vi "NOT4.vi"(1 "A":bool[](array[boolean])=[FALSE, FALSE, FALSE, FALSE, FALSE, FALSE, FALSE, FALSE, FALSE, FALSE, FALSE, FALSE, FALSE, FALSE, FALSE, FALSE]) -> (0 "z":bool[](array[boolean]))   [LabVIEW 2012]
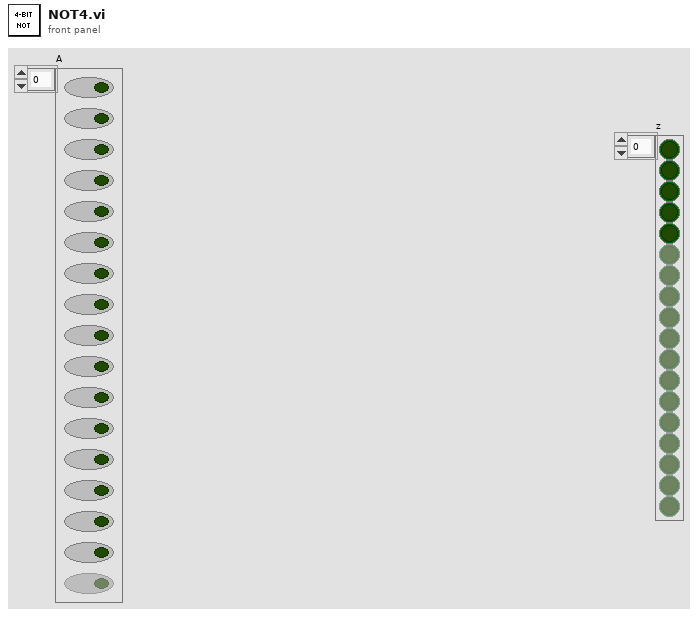
[diagram p1: front panel]
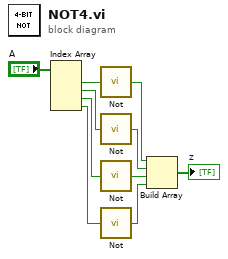
[diagram p0: block diagram]
diagram:
  n1 = Index Array(array="A") -> (element #1=w9:bool, element #2=w8:bool, element #3=w7:bool, element #4=w6:bool)  [unwired: 4 in]
  n2 = call "Not.vi"("In"=w9) -> ("Out"=w2:bool)
  n3 = call "Not.vi"("In"=w8) -> ("Out"=w3:bool)
  n4 = call "Not.vi"("In"=w7) -> ("Out"=w4:bool)
  n5 = call "Not.vi"("In"=w6) -> ("Out"=w5:bool)
  n6 = Build Array(w2, w3, w4, w5) -> (→"z":bool[])
